vi "Close Connection.vi"(8 "error in (no error)":errorcluster, 11 "NI-9381 (c series) in":refnum<class "NI-9381 (c series).lvclass">) -> (0 "error out":errorcluster, 3 "NI-9381 (c series) out":refnum<class "NI-9381 (c series).lvclass">)   [LabVIEW 2020, in "NI-9381 (c series).lvclass"]
uses:
  NI-9381 (c series).lvclass
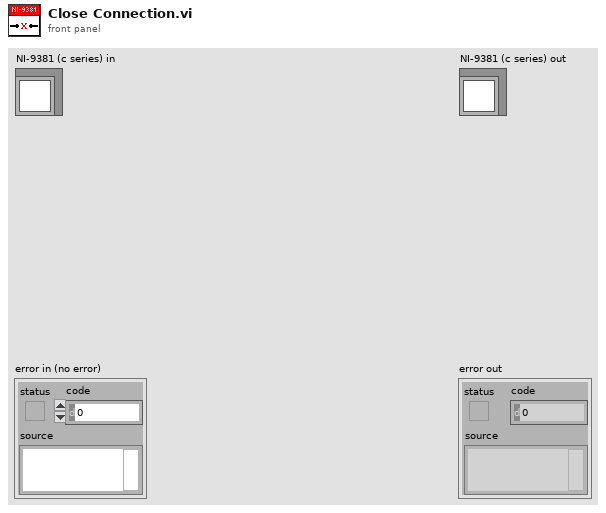
[diagram p1: front panel]
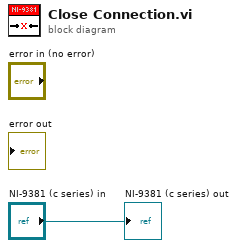
[diagram p0: block diagram]
diagram:
  "NI-9381 (c series) out" <- "NI-9381 (c series) in"
